vi "Word Easy Table (str).vi"(0 "report in":refnum<class "NI_report.lvclass">, 1 "auto format (none)":i32=-1, 2 "font settings source":u16(ring) items=["VI Inputs", "Font Dialog Box"], 5 "row headers":string[](array[string]), 7 "column headers":string[](array[string]), 9 "data":string[][](array[string]), 11 "error in (no error)":errorcluster, 12 "font":T1={"font name"="", "font size"=12.0, "bold"=2, "italic"=0, "underline"=0, "strike through"=0, "font color"=16777216} {"font size" format="%0.2f"; "strike through" items=["Unchanged", "Yes", "No"]; "underline" items=["Unchanged", "Yes", "No"]; "italic" items=["Unchanged", "Yes", "No"]; "bold" items=["Unchanged", "Yes", "No"]}) -> (4 "report out":refnum<class "NI_report.lvclass">, 6 "font out":T1={"font name"="", "font size"=0.0, "bold"=0, "italic"=0, "underline"=0, "strike through"=0, "font color"=16777216} {"font size" format="%0.2f"; "strike through" items=["Unchanged", "Yes", "No"]; "underline" items=["Unchanged", "Yes", "No"]; "italic" items=["Unchanged", "Yes", "No"]; "bold" items=["Unchanged", "Yes", "No"]}, 15 "error out":errorcluster)   [LabVIEW 2010, in "NI_ReportGenerationToolkit.lvlib"]
doc: "Inserts and formats a table into a Microsoft Word report. The data type you wire to the <B>data</B> input determines the polymorphic instance to use."
uses:
  <vilib>/addons/_office/NI_ReportGenerationToolkit.lvlib
  <vilib>/Utility/NIReport.llb/NI_report.lvclass
  <vilib>/addons/_office/_exclsub.llb/font.ctl
  <vilib>/Utility/NIReport.llb/Append Text Table to Report (wrap).vi
  <vilib>/Utility/NIReport.llb/Word/NI_Word.lvclass
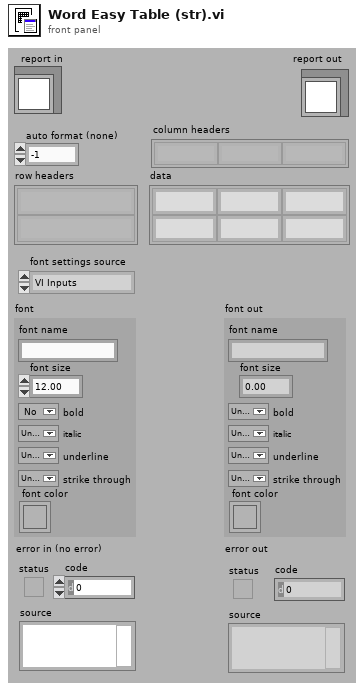
[diagram p1: front panel]
types:
  T1 = typedef "NI_ReportGenerationToolkit.lvlib/font.ctl" = cluster{"font name":string, "font size":dbl, "bold":u16, "italic":u16, "underline":u16, "strike through":u16, "font color":u32}
  T2 = cluster{"Charset (-1)":i16, "Weight (-1)":i16, "Name":string, "Size":string}
  T3 = cluster{i32, i32, i32, i32, "charset":i16, "weight":i16, "name":string, "size":string, "text color":u32}
  T4 = cluster{"italic":u16, "strike through":u16, "underline":u16, "bold":u16}
  T5 = typedef "NI_ReportGenerationCore.lvlib/font.ctl" = cluster{"font name":string, "font size":dbl, "bold":u16, "italic":u16, "underline":u16, "strike through":u16, "font color":u32}
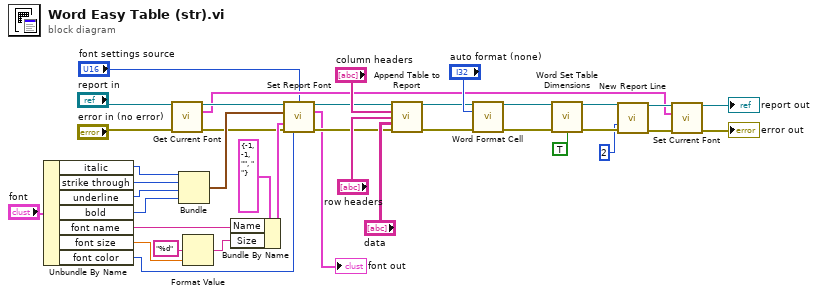
[diagram p0: block diagram]
diagram:
  n1 = Unbundle By Name("font") -> ("italic"=w21:u16, "strike through"=w20:u16, "underline"=w19:u16, "bold"=w18:u16, "font name"=w23:string, "font size"=w16:dbl, "font color"=w13:u32)
  n2 = call <vilib>:"Get Current Font.vi"("report in"="report in", "error in (no error)"="error in (no error)") -> ("report.lvclass"=w8:refnum<class "NI_report.lvclass">, "font"=w3:T3, "error out"=w9:errorcluster)  [unwired: 11 out]
  n3 = Bundle("italic"=w21, "strike through"=w20, "underline"=w19, "bold"=w18) -> (w12:T4)  [unwired: 1 out]
  n4 = Format Value(format string="%d", value (0)=w16) -> (output string=w15:string)  [unwired: 1 out]
  n5 = Bundle By Name(cluster=T2 {"Charset (-1)"=-1, "Weight (-1)"=-1, "Name"="", "Size"=" "} ("font settings"), "Name"=w23, "Size"=w15) -> (w14:T2)
  n6 = call-dynamic "Set Report Font.vi"("report in"=w8, "text color (unchanged)"=w13, "font settings source"="font settings source", "text options"=w12, "font settings"=w14, "error in (no error)"=w9) -> ("report out"=w25:refnum<class "NI_report.lvclass">, "font out"=→"font out":T5, "error out"=w26:errorcluster)  [unwired: 7 in]
  n7 = call-poly <vilib>:"Append Table to Report.vi"("report in"=w25, "column headers"="column headers", "row headers"="row headers", "text data"="data", "error in (no error)"=w26) -> ("report out"=w31:refnum<class "NI_report.lvclass">, "error out"=w30:errorcluster)  [unwired: 4 in, 5 out]
  n8 = call <vilib>:"Word Format Cell.vi"("report in"=w31, "autoformat (-1: none)"="auto format (none)", "error in (no error)"=w30) -> ("report out"=w33:refnum<class "NI_report.lvclass">, "error out"=w32:errorcluster)  [unwired: 4 in, 7 out]
  n9 = call <vilib>:"Word Set Table Dimensions.vi"("report in"=w33, "error in (no error)"=w32, "fit to page width? (F)"=TRUE ("fit to page width?")) -> ("report out"=w28:refnum<class "NI_report.lvclass">, "error out"=w29:errorcluster)  [unwired: 4 in, 7 out]
  n10 = call-dynamic "New Report Line.vi"("report in"=w28, "number of lines (1)"=2 ("number of lines"), "error in (no error)"=w29) -> ("report out"=w6:refnum<class "NI_report.lvclass">, "error out"=w7:errorcluster)  [unwired: 11 in]
  n11 = call <vilib>:"Set Current Font.vi"("report in"=w6, "font"=w3, "error in (no error)"=w7) -> ("report out"=→"report out":refnum<class "NI_report.lvclass">, "error out"=→"error out":errorcluster)  [unwired: 11 out]
